vi "曲线模型计算.vi"(11 "曲线模型":T1={"标液浓度1"=0.0, "测量吸光度1"=0.0, "样品1启用"=FALSE, "标液浓度2"=0.0, "测量吸光度2"=0.0, "样品2启用"=FALSE, "标液浓度3"=0.0, "测量吸光度3"=0.0, "样品3启用"=FALSE, "标液浓度4"=0.0, "测量吸光度4"=0.0, "样品4启用"=FALSE, "标液浓度5"=0.0, "测量吸光度5"=0.0, "样品5启用"=FALSE, "模型"=enum."线性", "精度"=4.0, "XY图"=[], "拟合公式"="", "r^2"=0.0, "标样一校准时间"=timestamp(0 s since 1904-01-01), "标样二校准时间"=timestamp(0 s since 1904-01-01), "标样三校准时间"=timestamp(0 s since 1904-01-01), "标样四校准时间"=timestamp(0 s since 1904-01-01), "标样五校准时间"=timestamp(0 s since 1904-01-01), "二次方程"={"c"=0.0, "x"=0.0, "x^2"=0.0}, "标定时间"=timestamp(0 s since 1904-01-01)} {"标定时间" format="%<%y/%m/%d %H:%M:%S>T"; "标样五校准时间" format="%<%y/%m/%d %H:%M:%S>T"; "标样四校准时间" format="%<%y/%m/%d %H:%M:%S>T"; "标样三校准时间" format="%<%y/%m/%d %H:%M:%S>T"; "标样二校准时间" format="%<%y/%m/%d %H:%M:%S>T"; "标样一校准时间" format="%<%y/%m/%d %H:%M:%S>T"; "r^2" format="%.7f"; "测量吸光度5" format="%#.6f"; "测量吸光度4" format="%#.6f"; "测量吸光度3" format="%#.6f"; "测量吸光度2" format="%#.6f"; "测量吸光度1" format="%#.6f"}) -> (3 "输出簇":T1)   [LabVIEW 2016, in "斯坦道总氮V2.lvlib"]
uses:
  <vilib>/Analysis/6fits.llb/Curve Fitting Criteria.ctl
  <vilib>/Analysis/NI_AALPro.lvlib
panel:
  # "校准时间"
  # "标液浓度"
  # "吸光值"
  # "空白"
  # "标样一"
  # "标样二"
  # "零点"
  # "跨度"
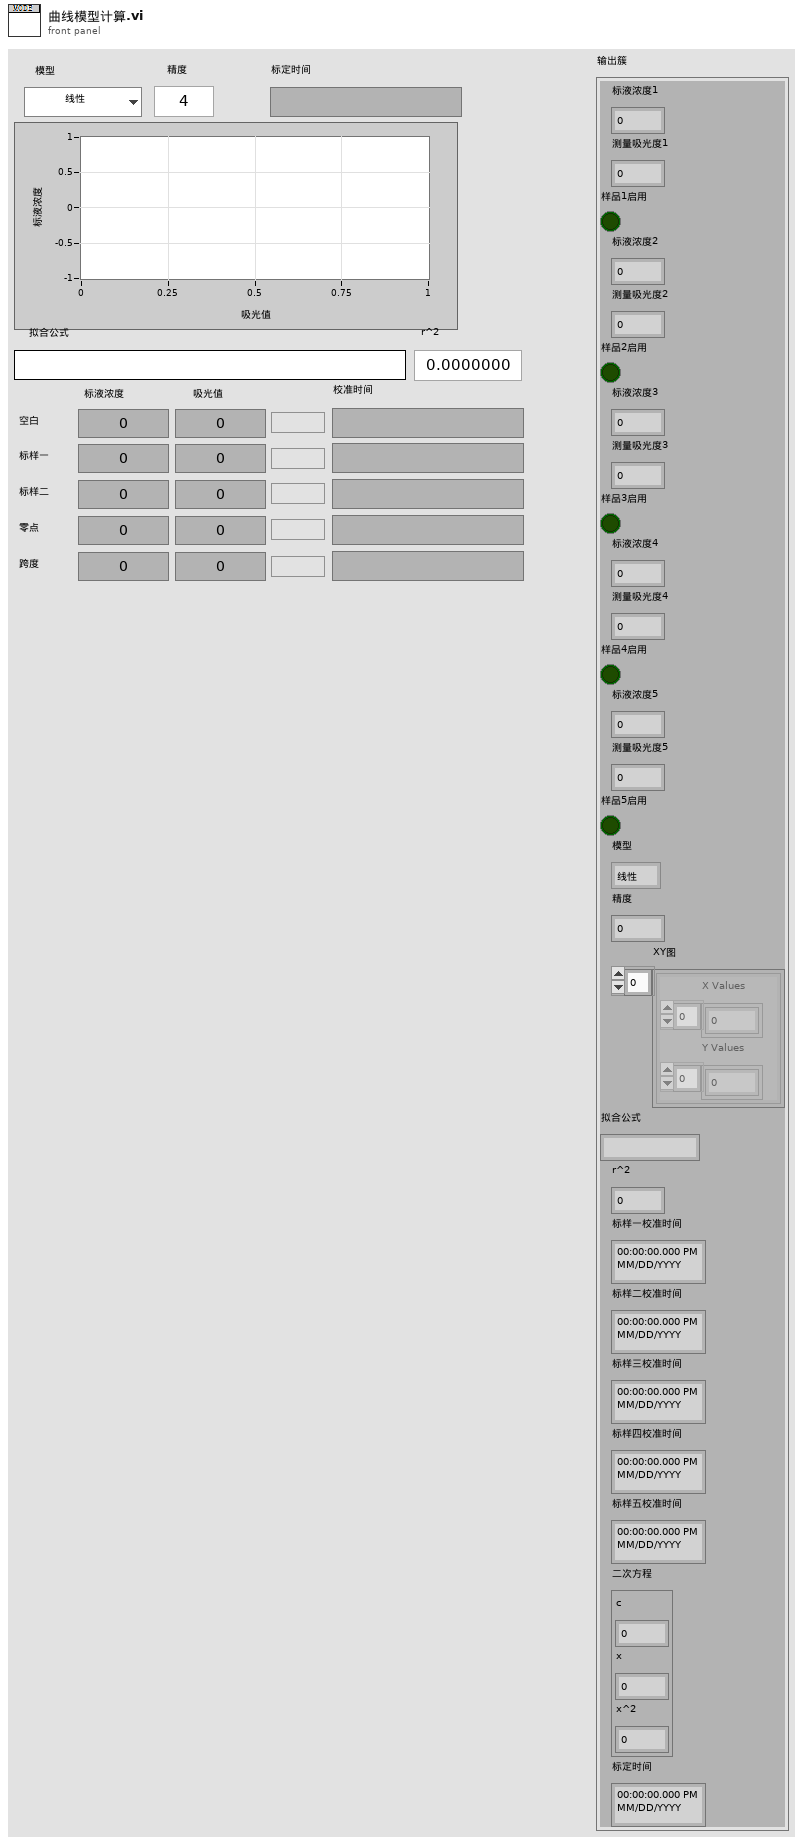
[diagram p1: front panel]
types:
  T1 = cluster{"标液浓度1":dbl, "测量吸光度1":dbl, "样品1启用":bool, "标液浓度2":dbl, "测量吸光度2":dbl, "样品2启用":bool, "标液浓度3":dbl, "测量吸光度3":dbl, "样品3启用":bool, "标液浓度4":dbl, "测量吸光度4":dbl, "样品4启用":bool, "标液浓度5":dbl, "测量吸光度5":dbl, "样品5启用":bool, "模型":enum32{"线性", "多项式"}, "精度":dbl, "XY图":cluster{"X Values":dbl[], "Y Values":dbl[]}[], "拟合公式":string, "r^2":dbl, "标样一校准时间":timestamp, "标样二校准时间":timestamp, "标样三校准时间":timestamp, "标样四校准时间":timestamp, "标样五校准时间":timestamp, "二次方程":cluster{"c":dbl, "x":dbl, "x^2":dbl}, "标定时间":timestamp}
  T2 = typedef "NI_AALPro.lvlib/Curve Fitting Criteria.ctl" = u16
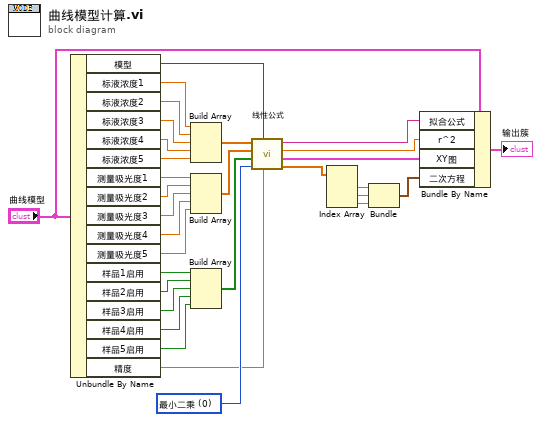
[diagram p0: block diagram]
diagram:
  w13 = T2 0 items=["最小二乘", "最小绝对残差", "Bisquare"] ("method")
  n1 = Unbundle By Name("曲线模型") -> ("模型"=w12:enum32{"线性", "多项式"}, "标液浓度1"=w31:dbl, "标液浓度2"=w30:dbl, "标液浓度3"=w29:dbl, "标液浓度4"=w28:dbl, "标液浓度5"=w27:dbl, "测量吸光度1"=w25:dbl, "测量吸光度2"=w24:dbl, "测量吸光度3"=w23:dbl, "测量吸光度4"=w22:dbl, "测量吸光度5"=w21:dbl, "样品1启用"=w19:bool, "样品2启用"=w18:bool, "样品3启用"=w17:bool, "样品4启用"=w16:bool, "样品5启用"=w15:bool, "精度"=w11:dbl)
  n2 = Build Array(w31, w30, w29, w28, w27) -> (w26:dbl[])
  n3 = Build Array(w25, w24, w23, w22, w21) -> (w20:dbl[])
  n4 = Build Array(w19, w18, w17, w16, w15) -> (w14:bool[])
  n5 = call "线性公式.vi"("精度"=w11, "模型"=w12, "method"=w13, "启用"=w14, "监测浓度"=w20, "标液浓度"=w26) -> ("Polynomial Coefficients 2"=w3:dbl[], "XY图"=w7:cluster{"X Values":dbl[], "Y Values":dbl[]}[], "r^2"=w8:dbl, "拟合方程"=w9:string)  [unwired: 2 in]
  n6 = Index Array(array=w3) -> (element #1=w6:dbl, element #2=w5:dbl, element #3=w4:dbl)  [unwired: 3 in]
  n7 = Bundle("slope"=w6, "slope"=w5, "slope"=w4) -> (w2:cluster{"slope":dbl, "slope":dbl, "slope":dbl})  [unwired: 1 in]
  n8 = Bundle By Name(cluster="曲线模型", "拟合公式"=w9, "r^2"=w8, "XY图"=w7, "二次方程"=w2) -> (→"输出簇":T1)
